vi "AVI U16 write-read multi frame.vi"() -> ()   [LabVIEW 2017]
doc: "This is a complete example on how to generate an AVI file from a set of 16bit (U16 or lower resolution) images/frames and read them back from the AVI file. Note that this will not work if you feed U32 data to the ArrayToColorImage vi."
panel:
  out "Average frame-read rate (fps)":u16
  in  "# frames":i32=100
  in  "Input data type":T1(ring)
  out "Average frame-write rate (fps)":u16
  out "Number of frames":i32
  in  "Image Pixels (I16)":i16[][][](array[numeric])=array7x512x512[1835008 elements]
  out "First I16 Image":T2(plugin-control)
  out "OK":bool
  out "Data read back (I16)":i16[][][](array[numeric])
  out "Last RGB Image":T2(plugin-control)
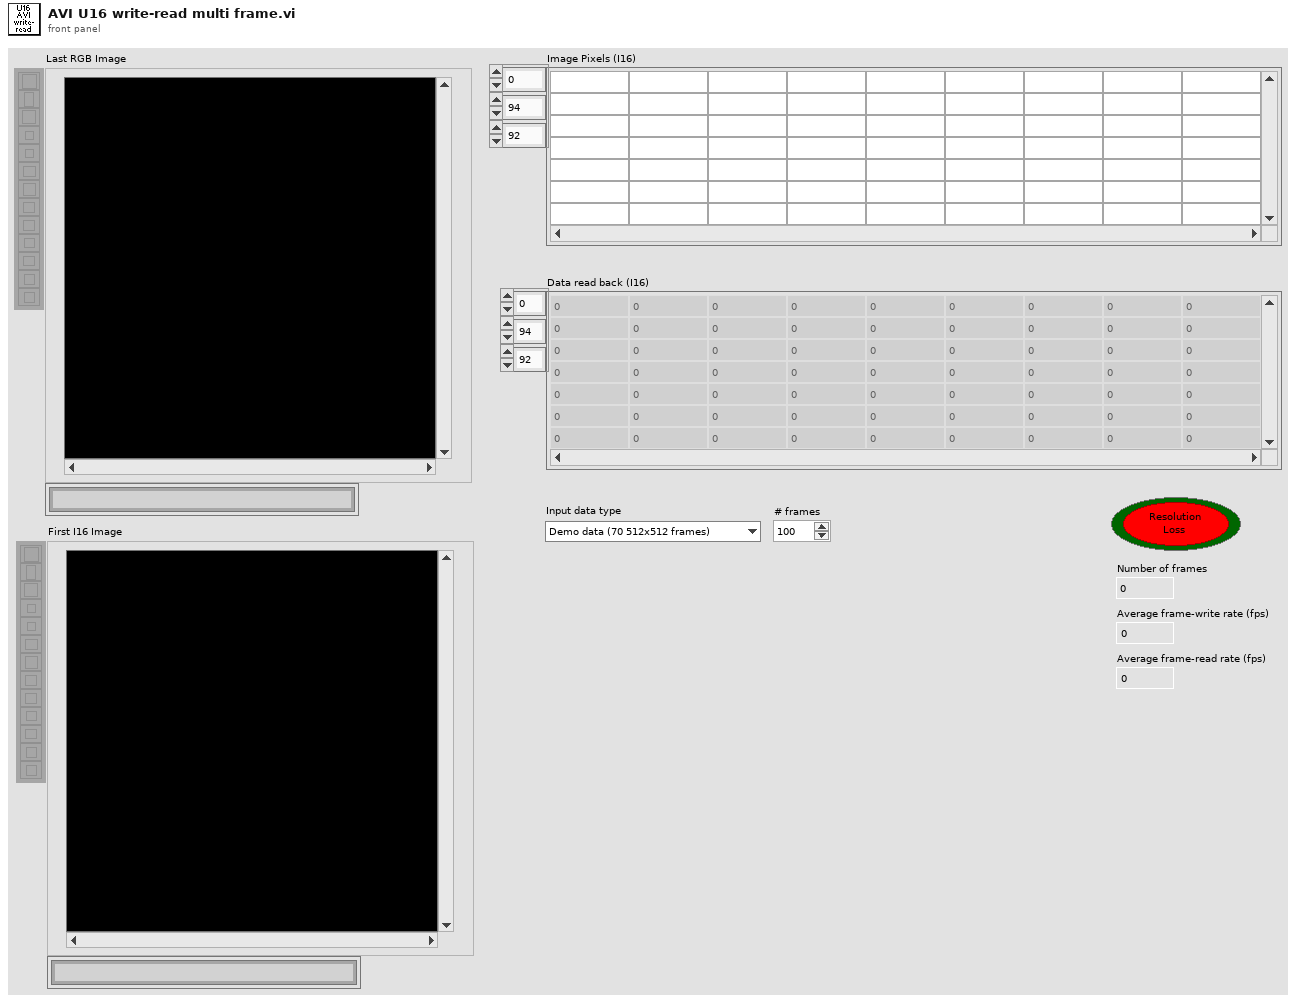
[diagram p1: front panel]
types:
  T1 = enum16{"Demo data (70 512x512 frames)", "100x100", "200x200", "512x512"}
  T2 = typedef "IMAQ Image.ctl" = refnum<image>
  T3 = typedef "Image Type" = u32
  T4 = typedef "IMAQ AVI2 Refnum.ctl" = refnum<k20>
  T5 = typedef "AviRefnum.ctl" = refnum<k1>
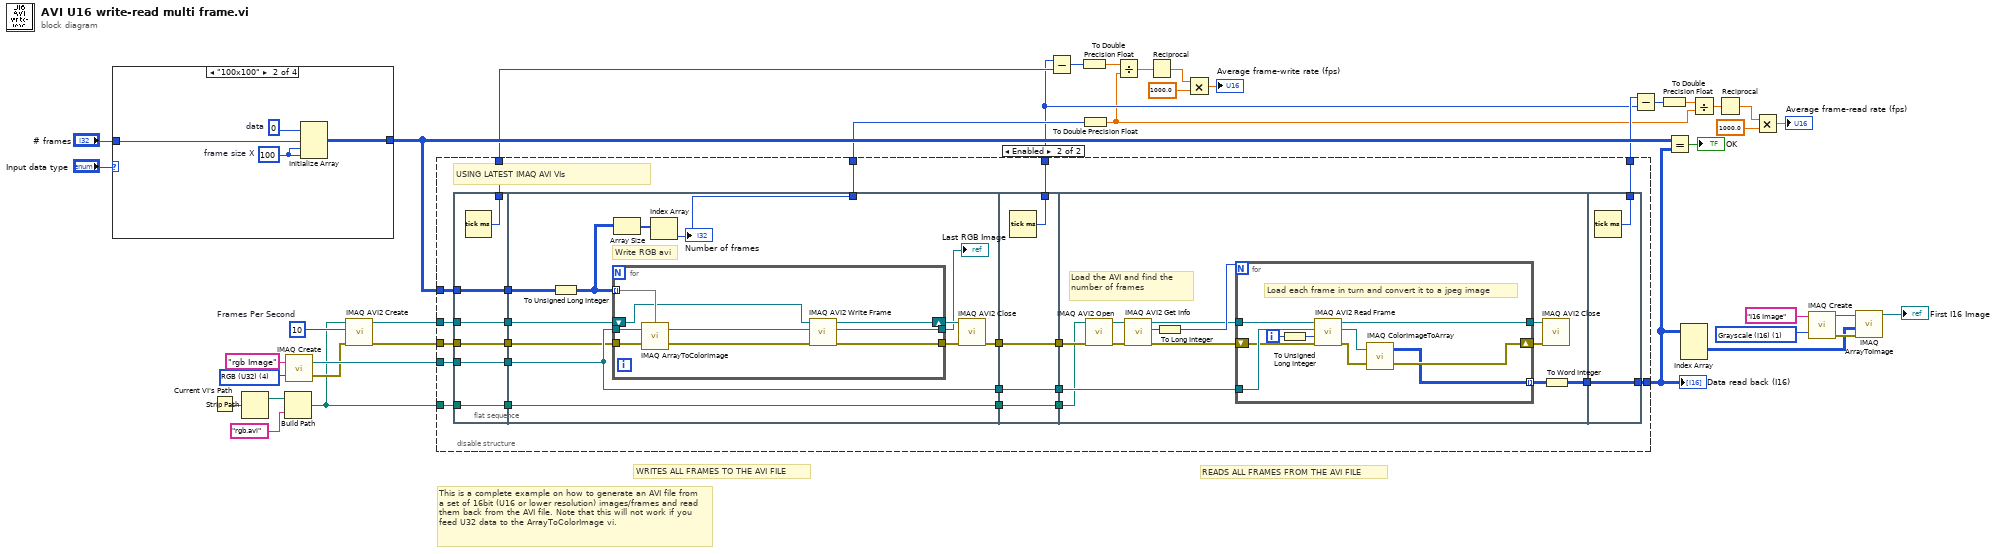
[diagram p0: block diagram]
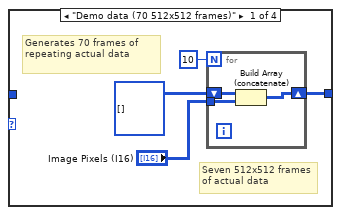
[diagram p2: hidden frame]
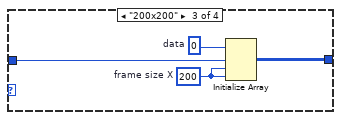
[diagram p3: hidden frame]
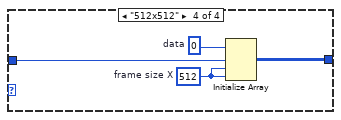
[diagram p4: hidden frame]
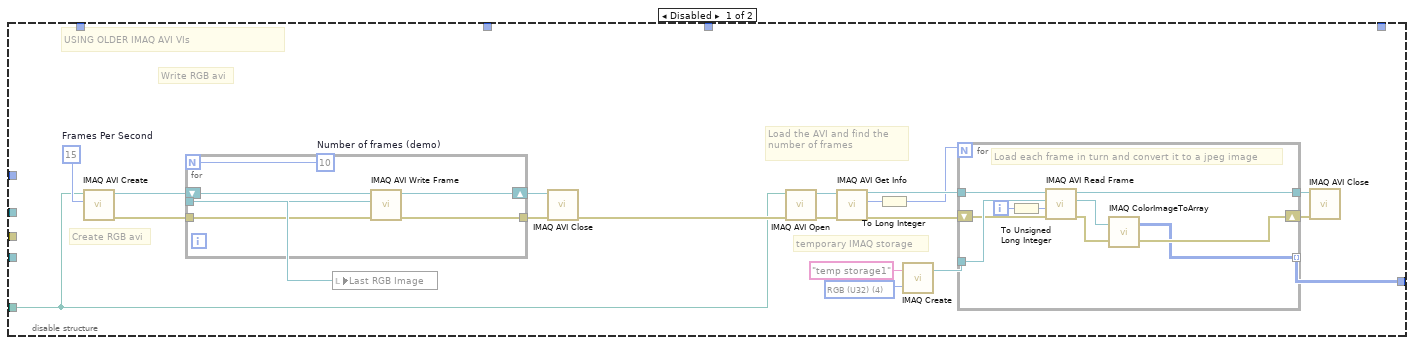
[diagram p5: hidden frame]
diagram:
  w20 = u32 10  # Frames Per Second
  w32 = T3 1 items=["Grayscale (U8)", "Grayscale (I16)", "Grayscale (SGL)", "Complex (CSG)", "RGB (U32)", "HSL (U32)", "RGB (U64)", "Grayscale (U16)"] ("Image Type")
  w36 = T3 4 items=["Grayscale (U8)", "Grayscale (I16)", "Grayscale (SGL)", "Complex (CSG)", "RGB (U32)", "HSL (U32)", "RGB (U64)", "Grayscale (U16)"] ("Image Type")
  # "This is a complete example on how to generate an AVI file from a set of 16bit (U16 or lower resolution) images/frames and read them back from the AVI file. Note that this will not work if you feed U32 data to the ArrayToColorImage vi."
  # "WRITES ALL FRAMES TO THE AVI FILE"
  # "READS ALL FRAMES FROM THE AVI FILE"
  n1 = case shown="\"100x100\"" "Input data type" {
    tunnel: [w40 w48 w52 w56] -> w26
    tunnel: "# frames" -> [_ w47 w51 w55]
    frame "Demo data (70 512x512 frames)" {
      # "Generates 70 frames of repeating actual data"
      # "Seven 512x512 frames\nof actual data"
      n2 = for {
        N: 10 -> [_]
        tunnel: "Image Pixels (I16)" -> [w45]
        shift-right: [w44] -> w40
        shift-left: i16[][][] [] ("Image Pixels (I16)") -> [w46]
        n3 = Build Array (concatenate)(w46, w45) -> (w44:i16[][][])
      }
    }
    frame "100x100" {
      w49 = 100  # frame size X
      w50 = i16 0  # data
      n4 = Initialize Array(w50, w47, w49, w49) -> (w48:i16[][][])
    }
    frame "200x200" {
      w53 = 200  # frame size X
      w54 = i16 0  # data
      n5 = Initialize Array(w54, w51, w53, w53) -> (w52:i16[][][])
    }
    frame "512x512" {
      w57 = 512  # frame size X
      w58 = i16 0  # data
      n6 = Initialize Array(w58, w55, w57, w57) -> (w56:i16[][][])
    }
  }
  n7 = Current VI's Path() -> (path=w39:path)
  n8 = Strip Path(path=w39) -> (stripped path=w38:path)  [unwired: 1 out]
  n9 = Build Path(base path=w38, name or relative path="rgb.avi") -> (appended path=w14:path)
  n10 = call "IMAQ Create"("Image Name"="rgb Image", "Image Type"=w36) -> ("New Image"=w29:T2, "error out"=w19:errorcluster)  [unwired: 2 in, 1 out]
  n11 = call "IMAQ AVI2 Create"("error in (no error)"=w19, "Frames Per Second"=w20, "AVI Path"=w14) -> ("error out"=w17:errorcluster, "AVI Refnum"=w18:T4)  [unwired: 7 in]
  n12 = disable-structure shown="Enabled" {
    disable-tunnel: w14 -> [w63 w117]
    disable-tunnel: [w62 w114] -> w28
    disable-tunnel: w29 -> [_ w115]
    disable-tunnel: w26 -> [_ w116]
    disable-tunnel: w18 -> [_ w107]
    disable-tunnel: w17 -> [_ w106]
    disable-tunnel: [_ w100] -> w4
    disable-tunnel: [_ w99] -> w16
    disable-tunnel: [_ w98] -> w15
    disable-tunnel: [_ w96] -> w5
    frame Disabled {
      w70 = T3 4 items=["Grayscale (U8)", "Grayscale (I16)", "Grayscale (SGL)", "Complex (CSG)", "RGB (U32)", "HSL (U32)", "RGB (U64)", "Grayscale (U16)"] ("Image Type")
      w76 = 10  # Number of frames (demo)
      w75 = u32 15  # Frames Per Second
      # "USING OLDER IMAQ AVI VIs"
      # "temporary IMAQ storage"
      # "Load the AVI and find the number of frames"
      # "Write RGB avi"
      # "Create RGB avi"
      n13 = call "IMAQ AVI Create"("Frames Per Second"=w75, "AVI Path"=w63) -> ("error out"=w79:errorcluster, "Avi Refnum"=w77:T5, "error in (no error)"=w61:errorcluster)  [unwired: 4 in, 3 out]
      n14 = for {
        N: w76 -> [_]
        shift-right: [w94] -> w78
        shift-left: w77 -> [w95]
        tunnel: [w93] -> w59
        tunnel: w79 -> [w92]
        tunnel: [w91] -> w80
        n15 = call "IMAQ AVI Write Frame"("error in (no error)"=w92, "Image"=w93, "Avi Refnum"=w95) -> ("error out"=w91:errorcluster, "Avi Refnum (duplicate)"=w94:T5)  [unwired: 1 in, 6 out]
      }
      n16 = local write "Last RGB Image"(w59) -> ()
      n17 = call "IMAQ AVI Close"("error in (no error)"=w80, "Avi Refnum"=w78) -> ("error out"=w64:errorcluster)  [unwired: 9 out]
      n18 = call "IMAQ AVI Open"("error in (no error)"=w64, "AVI Path"=w63) -> ("error out"=w71:errorcluster, "Avi Refnum"=w66:T5)  [unwired: 8 out]
      n19 = call "IMAQ AVI Get Info"("error in (no error)"=w71, "Avi Refnum"=w66) -> ("error out"=w72:errorcluster, "Number of Frames"=w74:u32, "Avi Refnum (duplicate)"=w68:T5)  [unwired: 7 out]
      n20 = To Long Integer(number=w74) -> (32bit integer=w60:i32)
      n21 = call "IMAQ Create"("Image Name"="temp storage1", "Image Type"=w70) -> ("New Image"=w65:T2)  [unwired: 2 in, 2 out]
      n22 = for {
        N: w60 -> [_]
        tunnel: w65 -> [w89]
        tunnel: [w88] -> w67
        tunnel: w68 -> [w87]
        shift-right: [w83] -> w73
        shift-left: w72 -> [w86]
        tunnel: [w82] -> w62 mode=indexing
        i -> [w85]
        # "Load each frame in turn and convert it to a jpeg image"
        n23 = To Unsigned Long Integer(number=w85) -> (unsigned 32bit integer=w81:u32)
        n24 = call "IMAQ AVI Read Frame"("error in (no error)"=w86, "Frame Number"=w81, "Image"=w89, "Avi Refnum"=w87) -> ("error out"=w84:errorcluster, "Image Out"=w90:T2, "Avi Refnum (duplicate)"=w88:T5)  [unwired: 1 in, 4 out]
        n25 = call "IMAQ ColorImageToArray"("Image"=w90, "error in (no error)"=w84) -> ("Image Pixels (U32)"=w82:u32[][], "error out"=w83:errorcluster)  [unwired: 1 in, 2 out]
      }
      n26 = call "IMAQ AVI Close"("error in (no error)"=w73, "Avi Refnum"=w67) -> ()  [unwired: 10 out]
    }
    frame Enabled {
      # "USING LATEST IMAQ AVI VIs"
      n27 = flat-sequence {
        tunnel: w106 -> [w119]
        tunnel: w107 -> [w120]
        tunnel: w115 -> [w121]
        tunnel: w116 -> [w122]
        tunnel: w117 -> [w123]
        tunnel: [w123] -> w105
        tunnel: [w122] -> w104
        tunnel: [w121] -> w103
        tunnel: [w120] -> w102
        tunnel: [w119] -> w101
        tunnel: [w118] -> w99
        tunnel: [w135] -> w113
        tunnel: [w128] -> w111
        tunnel: [w127] -> w109
        tunnel: w105 -> [w128]
        tunnel: w104 -> [w132]
        tunnel: w103 -> [w127]
        tunnel: w102 -> [w126]
        tunnel: w101 -> [w125]
        tunnel: [w124] -> w98
        tunnel: w113 -> [w148]
        tunnel: [w148] -> w112
        tunnel: w111 -> [w147]
        tunnel: [w147] -> w110
        tunnel: w109 -> [w146]
        tunnel: [w146] -> w108
        tunnel: [w145] -> w100
        tunnel: w112 -> [w152]
        tunnel: w110 -> [w150]
        tunnel: w108 -> [w151]
        tunnel: [w149] -> w97
        tunnel: [w173] -> w114
        tunnel: w97 -> [w173]
        tunnel: [w172] -> w96
        frame #0 {
          n28 = Tick Count (ms)() -> (millisecond timer value=w118:u32)
        }
        frame #1 {
          # "Write RGB avi"
          n29 = To Unsigned Long Integer(number=w132) -> (unsigned 32bit integer=w130:u32[][][])
          n30 = for {
            shift-right: [w144] -> w133
            shift-left: w126 -> [w137]
            tunnel: w125 -> [w141]
            tunnel: [w143] -> w134
            tunnel: w127 -> [w139]
            tunnel: w130 -> [w138] mode=indexing
            tunnel: [w136] -> w131
            n31 = call "IMAQ ArrayToColorImage"("Image Pixels (U32)"=w138, "Image"=w139, "error in (no error)"=w141) -> ("Image Out"=w140:T2, "error out"=w142:errorcluster)  [unwired: 1 in, 1 out]
            n32 = call "IMAQ AVI2 Write Frame"("error in (no error)"=w142, "Image"=w140, "AVI Refnum"=w137) -> ("error out"=w143:errorcluster, "Image Out (duplicate)"=w136:T2, "AVI Refnum (duplicate)"=w144:T4)  [unwired: 6 in]
          }
          "Last RGB Image" <- w131
          n33 = Array Size(array=w130) -> (size(s)=w129:i32[])
          n34 = Index Array(array=w129) -> (element=w124:i32)  [unwired: 1 in]
          "Number of frames" <- w124
          n35 = call "IMAQ AVI2 Close"("error in (no error)"=w134, "AVI Refnum"=w133) -> ("error out"=w135:errorcluster)  [unwired: 9 in]
        }
        frame #2 {
          n36 = Tick Count (ms)() -> (millisecond timer value=w145:u32)
        }
        frame #3 {
          # "Load the AVI and find the number of frames"
          n37 = call "IMAQ AVI2 Open"("error in (no error)"=w152, "AVI File Path"=w150) -> ("error out"=w160:errorcluster, "AVI Refnum"=w159:T4)  [unwired: 8 in]
          n38 = call "IMAQ AVI2 Get Info"("error in (no error)"=w160, "AVI Refnum"=w159) -> ("error out"=w157:errorcluster, "Number of Frames"=w158:u32, "AVI Refnum (duplicate)"=w155:T4)  [unwired: 5 in, 2 out]
          n39 = To Long Integer(number=w158) -> (32bit integer=w156:i32)
          n40 = for {
            N: w156 -> [_]
            tunnel: w151 -> [w166]
            tunnel: [w167] -> w154
            tunnel: w155 -> [w168]
            shift-right: [w170] -> w153
            shift-left: w157 -> [w163]
            tunnel: [w169] -> w161 mode=indexing
            i -> [w171]
            # "Load each frame in turn and convert it to a jpeg image"
            n41 = To Unsigned Long Integer(number=w171) -> (unsigned 32bit integer=w162:u32)
            n42 = call "IMAQ AVI2 Read Frame"("error in (no error)"=w163, "Frame Number"=w162, "Image"=w166, "AVI Refnum"=w168) -> ("error out"=w164:errorcluster, "Image Out"=w165:T2, "AVI Refnum (duplicate)"=w167:T4)  [unwired: 5 in]
            n43 = call "IMAQ ColorImageToArray"("Image"=w165, "error in (no error)"=w164) -> ("Image Pixels (U32)"=w169:u32[][], "error out"=w170:errorcluster)  [unwired: 1 in, 2 out]
          }
          n44 = call "IMAQ AVI2 Close"("error in (no error)"=w153, "AVI Refnum"=w154) -> ()  [unwired: 9 in, 1 out]
          n45 = To Word Integer(number=w161) -> (16bit integer=w149:i16[][][])
        }
        frame #4 {
          n46 = Tick Count (ms)() -> (millisecond timer value=w172:u32)
        }
      }
    }
  }
  "Data read back (I16)" <- w28
  n47 = Subtract(x=w4, y=w16) -> (x-y=w21:u32)
  n48 = To Double Precision Float(number=w21) -> (double precision float=w13:dbl)
  n49 = To Double Precision Float(number=w15) -> (double precision float=w3:dbl)
  n50 = Divide(x=w13, y=w3) -> (x/y=w23:dbl)
  n51 = Reciprocal(x=w23) -> (1/x=w24:dbl)
  n52 = Multiply(x=w24, y=1000.0) -> (x*y=→"Average frame-write rate (fps)":dbl)
  n53 = Subtract(x=w5, y=w4) -> (x-y=w9:u32)
  n54 = To Double Precision Float(number=w9) -> (double precision float=w10:dbl)
  n55 = Equal?(x=w26, y=w28) -> (x = y?=→"OK":bool)
  n56 = Index Array(array=w28) -> (element=w27:i16[][])  [unwired: 3 in]
  n57 = Divide(x=w10, y=w3) -> (x/y=w7:dbl)
  n58 = Reciprocal(x=w7) -> (1/x=w2:dbl)
  n59 = Multiply(x=w2, y=1000.0) -> (x*y=→"Average frame-read rate (fps)":dbl)
  n60 = call "IMAQ Create"("Image Name"="I16 Image", "Image Type"=w32) -> ("New Image"=w31:T2, "error out"=w30:errorcluster)  [unwired: 2 in, 1 out]
  n61 = call "IMAQ ArrayToImage"("error in (no error)"=w30, "Image Pixels (I16)"=w27, "Image"=w31) -> ("Image Out"=→"First I16 Image":T2)  [unwired: 7 in, 1 out]
